vi "Test Process Broadcast Lifecycle Changes.vi"(8 "error in (no error)":errorcluster, 11 "Process Test In":refnum<class "Process Test.lvclass">) -> (0 "error out":errorcluster, 3 "Process Test Out":refnum<class "Process Test.lvclass">)   [LabVIEW 2020, in "Process Test.lvclass"]
uses:
  Process Test.lvclass
  C:/Program Files (x86)/National Instruments/LabVIEW 2020/vi.lib/Asteme/LUnit/Test Case.lvclass
  <vilib>/Asteme/LUnit/Test Case.lvclass/Test Case.ctl
  <vilib>/Asteme/LUnit/LUnit Assertion Result.lvclass/LUnit Assertion Result.ctl
  Framework/Process/Process.lvclass/Process.ctl
  Support/Execution timer.vi
  <vilib>/Asteme/LUnit/Palette/Fail.vi
  <vilib>/Asteme/LUnit/Palette/Pass.vi
  <vilib>/Asteme/LUnit/Set Assertion Type.vi
  Framework/Process/Public/Lifecycle/Get Lifecycle State.vi
  Framework/Process/Private/SubVIs/Wait for finish.vi
  Framework/Process/Protected/Messaging/Enqueue Message.vi
  Framework/Process/Private/SubVIs/Set Lifecycle State.vi
  <vilib>/Asteme/LUnit/Add test result.vi
  <vilib>/Asteme/LUnit/LUnit Write Passed.vi
  <vilib>/Asteme/LUnit/LUnit Get Test Case.vi
  <vilib>/Asteme/LUnit/Assertion Result/LUnit Get Test Name.vi
  <vilib>/Asteme/LUnit/LUnit Write Message.vi
  <vilib>/Asteme/LUnit/LUnit Write Description.vi
  <vilib>/Asteme/LUnit/LUnit Write Assertion Type.vi
  <vilib>/Utility/error.llb/Clear Errors.vi
  <vilib>/Asteme/LUnit/Read Test Case Name.vi
  Support/Event Helpers/Dequeue Event Message.vi
  <vilib>/Utility/error.llb/Error Cluster From Error Code.vi
  <vilib>/Asteme/LUnit/LUnit Assertion Result.lvclass
  Framework/Process/Process.lvclass
  <vilib>/Asteme/LUnit/Test Case.lvclass
  Support/Event Helpers/Event Helpers.lvlib
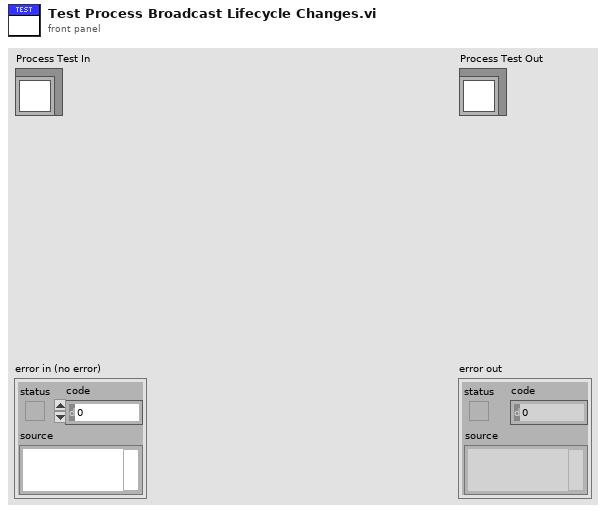
[diagram p1: front panel]
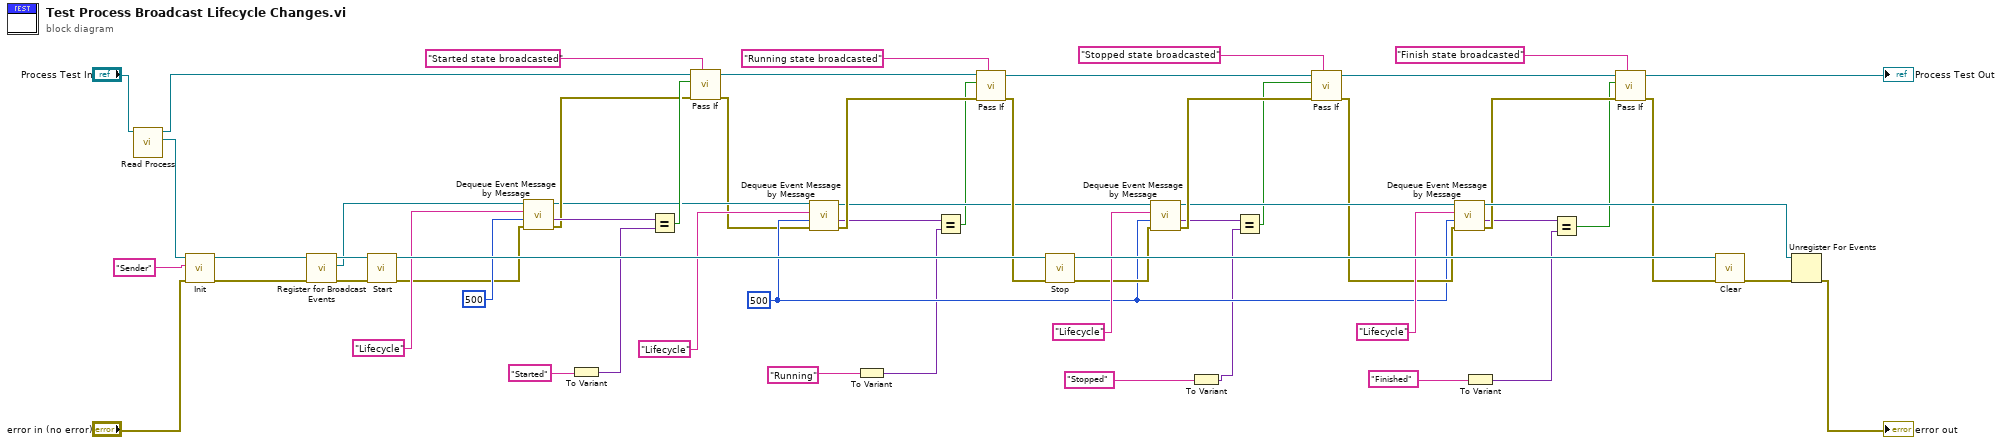
[diagram p0: block diagram]
diagram:
  w27 = 500
  n1 = call "Read Process.vi"("Process Test in"="Process Test In") -> ("Process.lvclass"=w51:refnum<class "Process.lvclass">, "Process Test out"=w6:refnum<class "Process Test.lvclass">)  [unwired: 8 in, 1 out]
  n2 = call-dynamic "Init.vi"("error in (no error)"="error in (no error)", "Name"="Sender" ("Message"), "Process In"=w51) -> ("error out"=w57:errorcluster, "Process Out"=w58:refnum<class "Process.lvclass">)  [unwired: 7 in]
  n3 = call "Register for Broadcast Events.vi"("error in (no error)"=w57, "Process In"=w58) -> ("error out"=w49:errorcluster, "Event Registration Refnum"=w10:refnum<event-registration>, "Process Out"=w50:refnum<class "Process.lvclass">)  [unwired: 7 in]
  n4 = call "Start.vi"("error in (no error)"=w49, "Process In"=w50) -> ("error out"=w8:errorcluster, "Process Out"=w48:refnum<class "Process.lvclass">)  [unwired: 8 in]
  n5 = call "Dequeue Event Message by Message.vi"("error in (no error)"=w8, "Timeout (-1)"=500, "Message"="Lifecycle", "Event Registration Refnum"=w10) -> ("error out"=w12:errorcluster, "Message Data"=w13:variant, "Event Registration Refnum Out"=w9:refnum<event-registration>)  [unwired: 3 in, 2 out]
  n6 = To Variant(anything="Started") -> (Variant=w17:variant)
  n7 = Equal?(x=w13, y=w17) -> (x = y?=w16:bool)
  n8 = call <vilib>:"Pass If.vi"("Description"="Started state broadcasted", "error in (no error)"=w12, "Pass?"=w16, "Test Case In"=w6) -> ("error out"=w7:errorcluster, "Test Case Out"=w5:refnum<class "Process Test.lvclass">)  [unwired: 6 in]
  n9 = call "Dequeue Event Message by Message.vi"("error in (no error)"=w7, "Timeout (-1)"=w27, "Message"="Lifecycle", "Event Registration Refnum"=w9) -> ("error out"=w46:errorcluster, "Message Data"=w44:variant, "Event Registration Refnum Out"=w31:refnum<event-registration>)  [unwired: 3 in, 2 out]
  n10 = To Variant(anything="Running" ("Message")) -> (Variant=w23:variant)
  n11 = Equal?(x=w44, y=w23) -> (x = y?=w24:bool)
  n12 = call <vilib>:"Pass If.vi"("Description"="Running state broadcasted", "error in (no error)"=w46, "Pass?"=w24, "Test Case In"=w5) -> ("error out"=w45:errorcluster, "Test Case Out"=w26:refnum<class "Process Test.lvclass">)  [unwired: 6 in]
  n13 = call "Stop.vi"("error in (no error)"=w45, "Process In"=w48) -> ("error out"=w29:errorcluster, "Process Out"=w56:refnum<class "Process.lvclass">)  [unwired: 7 in, 1 out]
  n14 = call "Dequeue Event Message by Message.vi"("error in (no error)"=w29, "Timeout (-1)"=w27, "Message"="Lifecycle", "Event Registration Refnum"=w31) -> ("error out"=w35:errorcluster, "Message Data"=w33:variant, "Event Registration Refnum Out"=w30:refnum<event-registration>)  [unwired: 3 in, 2 out]
  n15 = To Variant(anything="Stopped" ("Message")) -> (Variant=w21:variant)
  n16 = Equal?(x=w33, y=w21) -> (x = y?=w22:bool)
  n17 = call <vilib>:"Pass If.vi"("Description"="Stopped state broadcasted", "error in (no error)"=w35, "Pass?"=w22, "Test Case In"=w26) -> ("error out"=w28:errorcluster, "Test Case Out"=w25:refnum<class "Process Test.lvclass">)  [unwired: 6 in]
  n18 = call "Dequeue Event Message by Message.vi"("error in (no error)"=w28, "Timeout (-1)"=w27, "Message"="Lifecycle", "Event Registration Refnum"=w30) -> ("error out"=w37:errorcluster, "Message Data"=w20:variant, "Event Registration Refnum Out"=w43:refnum<event-registration>)  [unwired: 3 in, 2 out]
  n19 = To Variant(anything="Finished" ("Message")) -> (Variant=w19:variant)
  n20 = Equal?(x=w20, y=w19) -> (x = y?=w18:bool)
  n21 = call <vilib>:"Pass If.vi"("Description"="Finish state broadcasted", "error in (no error)"=w37, "Pass?"=w18, "Test Case In"=w25) -> ("error out"=w36:errorcluster, "Test Case Out"=→"Process Test Out":refnum<class "Process Test.lvclass">)  [unwired: 6 in]
  n22 = call-dynamic "Clear.vi"("error in (no error)"=w36, "Process In"=w56) -> ("error out"=w55:errorcluster)  [unwired: 8 in, 1 out]
  n23 = Unregister For Events(event registration refnum=w43, error in=w55) -> (error out=→"error out":errorcluster)
